vi "WPI_AnalogTriggerClose.vi"(8 "error in (no error)":errorcluster, 10 "Close Dependencies":bool=TRUE, 11 "AnalogTriggerDevRef":T1={"DevStatus"={"status"=FALSE, "code"=0, "source"=""}, "AnalogTriggerIndex"=enum."Invalid"}) -> (0 "error out":errorcluster)   [LabVIEW 2017]
doc: "Closes the reference to the analog trigger you specify. Use this VI to close each analog trigger reference that you open with the Open VI.\n\nThis software is licensed. Open the labview\\readme\\WPI Robotics Library Open Source License.txt file for more information."
uses:
  <vilib>/Rock Robotics/SystemInterfaces/AnalogTrigger/FPGA_AnalogTriggerDevRef.ctl
  <vilib>/Rock Robotics/SystemInterfaces/AnalogTrigger/FPGA_AnalogTriggerIndex.ctl
  <vilib>/Rock Robotics/WPI/AnalogChannel/WPI_AnalogChannelDevRef.ctl
  <vilib>/Rock Robotics/SystemInterfaces/AI/FPGA_AIChannel.ctl
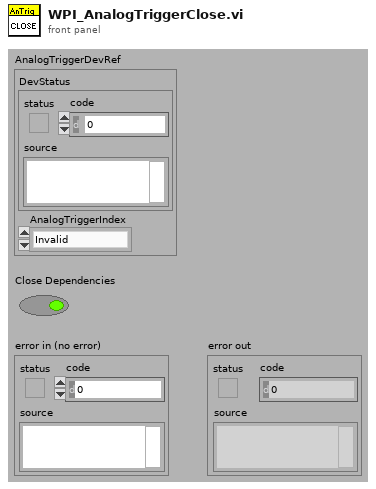
[diagram p1: front panel]
types:
  T1 = typedef "FPGA_AnalogTriggerDevRef.ctl" = cluster{"DevStatus":errorcluster, "AnalogTriggerIndex":T2}
  T2 = typedef "FPGA_AnalogTriggerIndex.ctl" = enum8{"Trig 0", "Trig 1", "Trig 2", "Trig 3", "Trig 4", "Trig 5", "Trig 6", "Trig 7", "Invalid"}
  T3 = typedef "WPI_AnalogChannelDevRef.ctl" = cluster{"DevStatus":errorcluster, "Analog Channel":T4}
  T4 = typedef "FPGA_AIChannel.ctl" = enum8{"AI 0", "AI 1", "AI 2", "AI 3", "AI MXP 0", "AI MXP 1", "AI MXP 2", "AI MXP 3", "Invalid"}
  T5 = typedef "FPGA_AnalogTriggerSource.ctl" = cluster{"Channel":T4, "Averaged":bool, "Filter":bool}
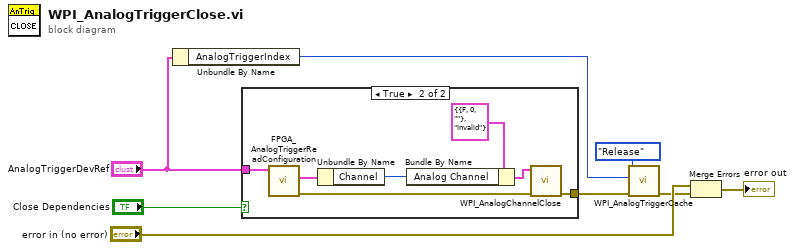
[diagram p0: block diagram]
diagram:
  n1 = Unbundle By Name("AnalogTriggerDevRef") -> ("AnalogTriggerIndex"=w4:T2)
  n2 = case shown="True" "Close Dependencies" {
    tunnel: [_ w14] -> w5
    tunnel: "AnalogTriggerDevRef" -> [_ w13]
    frame False {
    }
    frame True {
      n3 = call <vilib>:"FPGA_AnalogTriggerReadConfiguration.vi"("AnalogTriggerDevRef"=w13) -> ("error out"=w15:errorcluster, "AnalogTriggerSource"=w12:T5)  [unwired: 1 in, 8 out]
      n4 = Unbundle By Name(w12) -> ("Channel"=w9:T4)
      n5 = Bundle By Name(cluster=T3 {"DevStatus"={"status"=FALSE, "code"=0, "source"=""}, "Analog Channel"=enum."Invalid"} ("AIDeviceRef"), "Analog Channel"=w9) -> (w11:T3)
      n6 = call <vilib>:"WPI_AnalogChannelClose.vi"("error in (no error)"=w15, "AIDeviceRef"=w11) -> ("error out"=w14:errorcluster)  [unwired: 9 out]
    }
  }
  n7 = call <vilib>:"WPI_AnalogTriggerCache.vi"("error in (no error)"=w5, "AnalogTriggerToRelease"=w4, "Operation"=enum16{"Acquire", "Release"}."Release") -> ("error out"=w2:errorcluster)  [unwired: 8 out]
  n8 = Merge Errors("error in (no error)", w2) -> (→"error out":errorcluster)
